vi "onCreated.vi"(8 "error in (no error)":errorcluster, 11 "Edit":refnum<class "Edit.lvclass">) -> (0 "error out":errorcluster, 3 "Edit out":refnum<class "Edit.lvclass">)   [LabVIEW 2019, in "Edit.lvclass"]
uses:
  Edit.lvclass
  C:/Program Files (x86)/National Instruments/LabVIEW 2019/vi.lib/JKI/JKI SMO/SMO/SMO.lvclass
  <vilib>/JKI/JKI SMO/SMO/SMO.lvclass
panel:
  # "For instructions on how to use the JKI State Machine Objects, examples and video tutorials, visit:\nhttp://jki.net/state-machine-objects/\n\nJKI State Machine Objects™\nhttp://jki.net/state-machine-objects/\nCopyright (C) 2005-2015, JKI <info@jki.net>\nALL RIGHTS RESERVED"
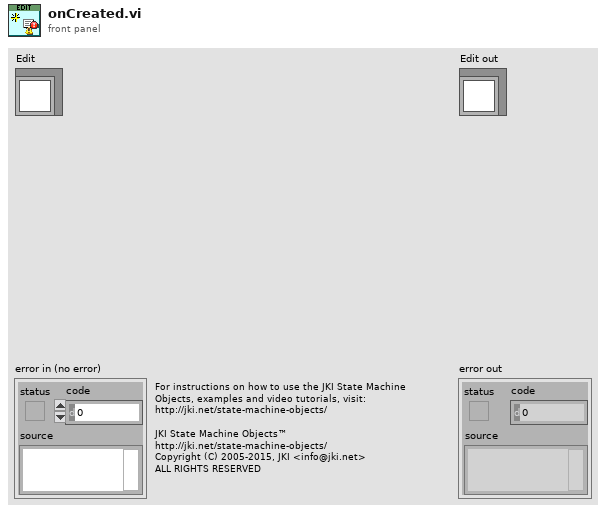
[diagram p1: front panel]
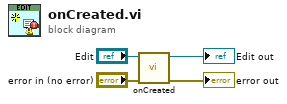
[diagram p0: block diagram]
diagram:
  n1 = call-parent "onCreated.vi"("error in (no error)"="error in (no error)", "SMO"="Edit") -> ("error out"=→"error out":errorcluster, "SMO out"=→"Edit out":refnum<class "Edit.lvclass">)  [unwired: 8 in]
